vi "lv-ros-bridge_write.vi"(8 "error in (no error)":errorcluster, 10 "rosbridge port":u16=9090, 11 "rosbridge server IP":string="192.168.5.103") -> (0 "error out":errorcluster)   [LabVIEW 2013]
uses:
  <vilib>/Intelligent Energy/WebSockets API/WebSockets/WebSockets.lvlib
panel:
  in  "advertise message":string="{\"op\":\"advertise\", \"topic\":\"rio/odom\",\"type\":\"sterowanie/velocities\"}"
  out "output cluster":T1
  in  "msg.vel5":i16
  in  "msg.vel4":i16
  in  "msg.vel3":i16
  in  "msg.vel2":i16
  in  "msg.vel1":i16
  in  "msg.vel0":i16
  in  "Topic to write":string="rio/odom"
  in  "outgoing message":T1
  out "raw frame":string
  in  "stop":bool
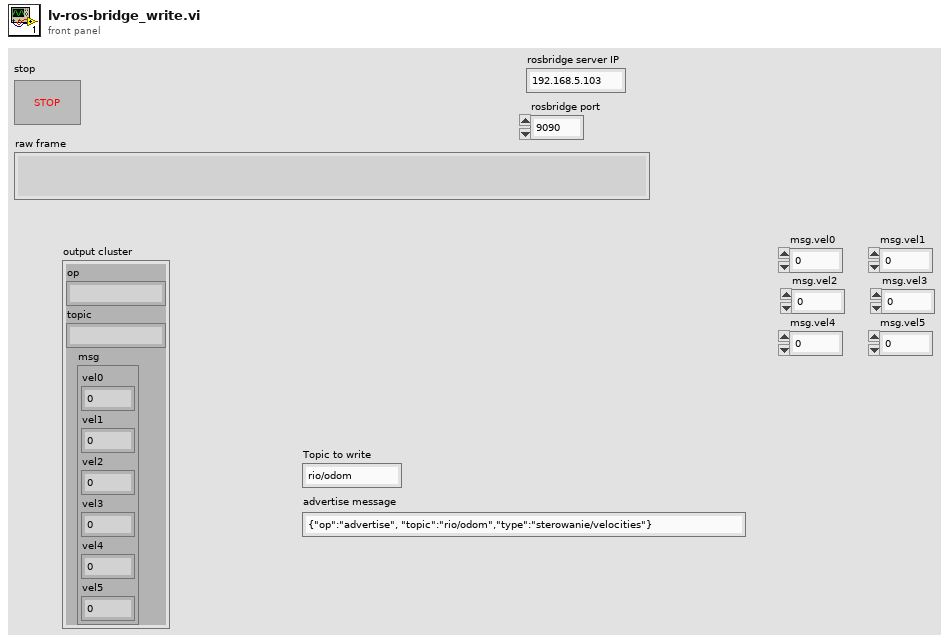
[diagram p1: front panel]
types:
  T1 = cluster{"op":string, "topic":string, "msg":cluster{"vel0":i16, "vel1":i16, "vel2":i16, "vel3":i16, "vel4":i16, "vel5":i16}}
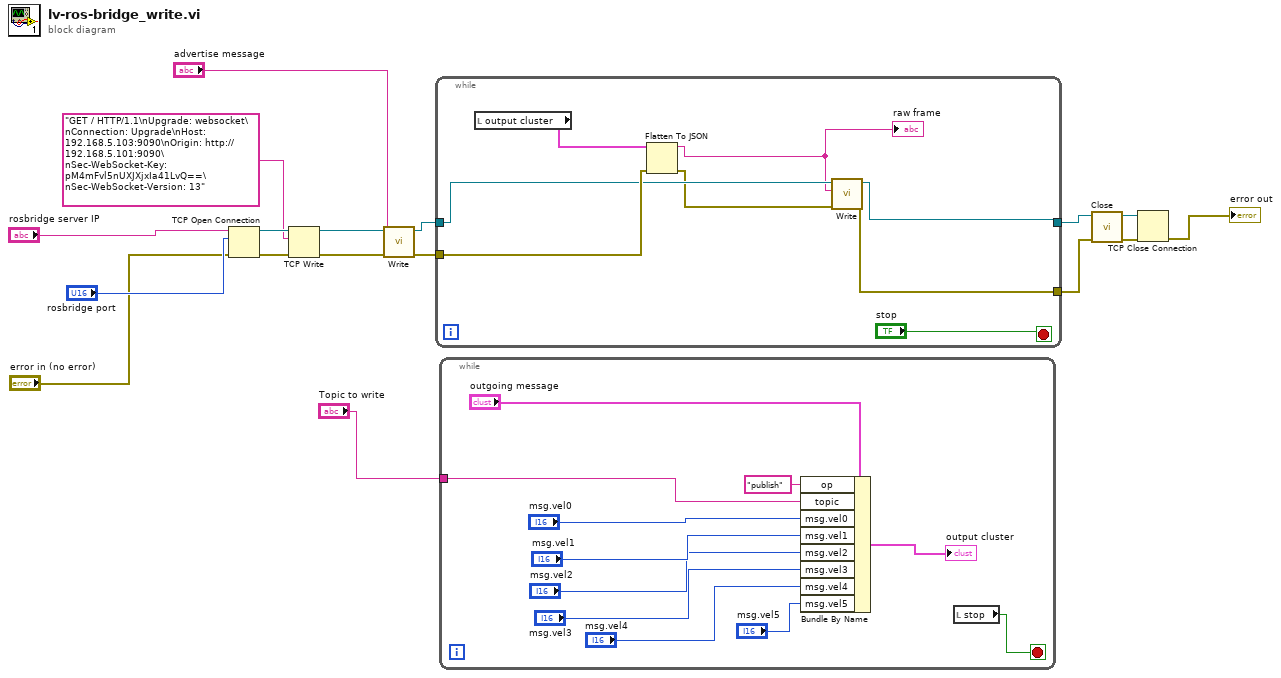
[diagram p0: block diagram]
diagram:
  n1 = TCP Open Connection(address="rosbridge server IP", remote port or service name="rosbridge port", error in (no error)="error in (no error)") -> (connection ID=w15:refnum<k5>, error out=w13:errorcluster)  [unwired: 2 in]
  n2 = TCP Write(connection ID=w15, data in="GET / HTTP/1.1\nUpgrade: websocket\nConnection: Upgrade\nHost: 192.168.5.103:9090\nOrigin: http://192.168.5.101:9090\nSec-WebSocket-Key: pM4mFvl5nUXJXjxIa41LvQ==\nSec-WebSocket-Version: 13", error in (no error)=w13) -> (connection ID out=w2:refnum<k5>, error out=w1:errorcluster)  [unwired: 1 in, 1 out]
  n3 = call <vilib>:"Write.vi"("error in (no error)"=w1, "Data"="advertise message", "WebSocket Connection in"=w2) -> ("error out"=w5:errorcluster, "WebSocket Connection out"=w4:refnum<k5>)  [unwired: 7 in]
  n4 = while {
    tunnel: [w22] -> w10
    tunnel: [w21] -> w9
    tunnel: w4 -> [w23]
    tunnel: w5 -> [w24]
    stop <- "stop" stop-if-true
    n5 = local read "output cluster"() -> (w25:T1)
    n6 = Flatten To JSON(anything=w25, error in (no error)=w24) -> (JSON string=w18:string, 11:w20:errorcluster)  [unwired: 1 in]
    "raw frame" <- w18
    n7 = call <vilib>:"Write.vi"("error in (no error)"=w20, "Data"=w18, "WebSocket Connection in"=w23) -> ("error out"=w21:errorcluster, "WebSocket Connection out"=w22:refnum<k5>)  [unwired: 7 in]
  }
  n8 = while {
    tunnel: "Topic to write" -> [w35]
    stop <- w27 stop-if-true
    n9 = Bundle By Name(cluster="outgoing message", "op"="publish", "topic"=w35, "msg.vel0"="msg.vel0", "msg.vel1"="msg.vel1", "msg.vel2"="msg.vel2", "msg.vel3"="msg.vel3", "msg.vel4"="msg.vel4", "msg.vel5"="msg.vel5") -> (→"output cluster":T1)
    n10 = local read "stop"() -> (w27:bool)
  }
  n11 = call <vilib>:"Close.vi"("error in (no error)"=w9, "WebSocket Connection in"=w10) -> ("error out"=w11:errorcluster, "WebSocket Connection in"=w12:refnum<k5>)  [unwired: 8 in]
  n12 = TCP Close Connection(connection ID=w12, error in (no error)=w11) -> (error out=→"error out":errorcluster)  [unwired: 1 in, 1 out]
